vi "Instrument.MessageFromProcess.EventStructure.vi"(6 "timeout (ms) [500]":i32, 8 "error in (no error)":errorcluster, 11 "Event Registration Refnum in":refnum<event-registration>) -> (0 "error out":errorcluster, 1 "Data":variant, 2 "Command":string, 3 "Event Registration Refnum out":refnum<event-registration>, 4 "ID":string)   [LabVIEW 2019, in "Instrument.lvclass"]
uses:
  Instrument.lvclass
  Typedefs/PublicEvents--Instrument.MessageFromProcess.ctl
  <userlib>/LevyLab/RemoteControl/Typedefs/Message--Cluster.ctl
  <userlib>/LevyLab/RemoteControl/RemoteControl.lvclass
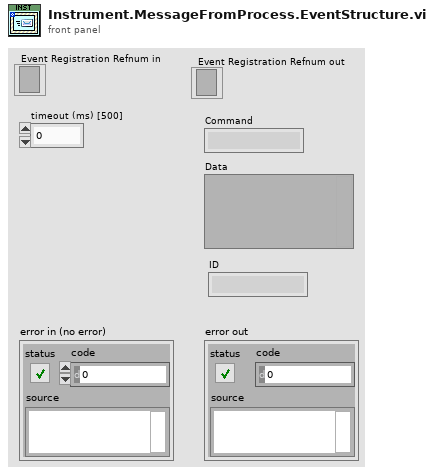
[diagram p1: front panel]
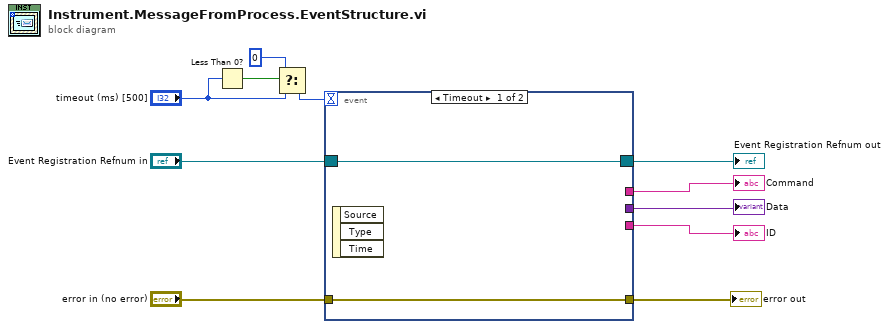
[diagram p0: block diagram]
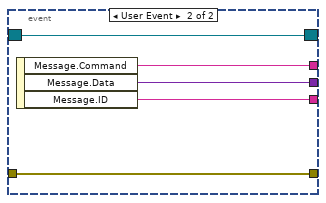
[diagram p2: hidden frame]
diagram:
  n1 = Less Than 0?(x="timeout (ms) [500]") -> (x < 0?=w4:bool)
  n2 = Select(t=0, s=w4, f="timeout (ms) [500]") -> (s? t:f=w2:i32)
  n3 = event shown="[0] Timeout" {
    selector: "Event Registration Refnum in" -> [w12 w14]
    dyn-events: [w12 w14] -> w5
    timeout: w2 -> [_ _]
    tunnel: [_ w18] -> w7
    tunnel: [_ w17] -> w8
    tunnel: [_ w16] -> w9
    tunnel: "error in (no error)" -> [w13 w15]
    tunnel: [w13 w15] -> w11
    event Timeout {
      n4 = event-data() -> ()  [unwired: 1 in, 3 out]
    }
    event User Event {
      n5 = event-data() -> ("Message.Command"=w18:string, "Message.Data"=w17:variant, "Message.ID"=w16:string)  [unwired: 1 in]
    }
  }
  "error out" <- w11
  "ID" <- w9
  "Data" <- w8
  "Command" <- w7
  "Event Registration Refnum out" <- w5
